vi "Utility Format Flow Rate.vi"(8 "error in (no error)":errorcluster, 11 "Flow Rate":dbl) -> (0 "error out":errorcluster, 3 "Formatted Flow Rate":string)   [LabVIEW 2020, in "ChromTech Series I Drivers.lvlib"]
uses:
  <instrlib>/RxnRover/ChromtechSeriesIDriver/ChromTech Series I Drivers.lvlib
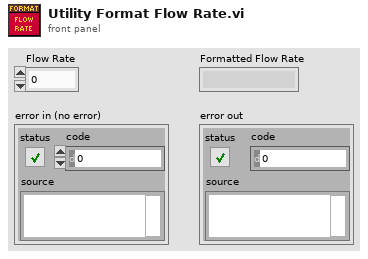
[diagram p1: front panel]
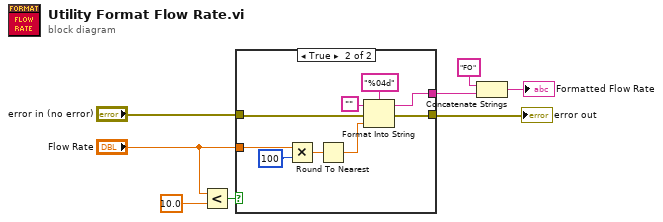
[diagram p0: block diagram]
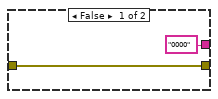
[diagram p2: hidden frame]
diagram:
  n1 = Less?(x="Flow Rate", y=10.0) -> (x < y?=w6:bool)
  n2 = case shown="True" w6 {
    tunnel: "error in (no error)" -> [w10 w18]
    tunnel: "Flow Rate" -> [_ w14]
    tunnel: [w10 w17] -> w5
    tunnel: ["0000" w16] -> w1
    frame False {
    }
    frame True {
      n3 = Multiply(x=w14, y=100) -> (x*y=w13:dbl)
      n4 = Round To Nearest(number=w13) -> (nearest integer value=w11:dbl)
      n5 = Format Into String(format string="%04d", initial string="", error in=w18, w11) -> (resulting string=w16:string, error out=w17:errorcluster)
    }
  }
  "error out" <- w5
  n6 = Concatenate Strings("FO", w1) -> (→"Formatted Flow Rate":string)
